vi "ToTable.vi"(8 "error in":errorcluster, 9 "Table Index (0)":i32, 10 "variant":variant, 11 "Sequencer Module editor node in":refnum<class "Sequencer Module editor node.lvclass">) -> (0 "error out":errorcluster, 1 "row headers":string[](array[string]), 2 "table":string[][](array[string]), 3 "Sequencer Module editor node out":refnum<class "Sequencer Module editor node.lvclass">)   [LabVIEW 2015, in "Sequencer Module editor node.lvclass"]
doc: "Generates the strings needed to display on a table based on the information found in the engine and module configuration classes."
uses:
  Sequencer Module editor node.lvclass
  module/configuration/Sequencer Module configuration.lvclass
  <vilib>/NI/Module Execution Interface/Engine Configuration/engine configuration.lvclass
  <vilib>/NI/DCAF/Tag Editor Core/control module/editor node/control module editor.lvclass
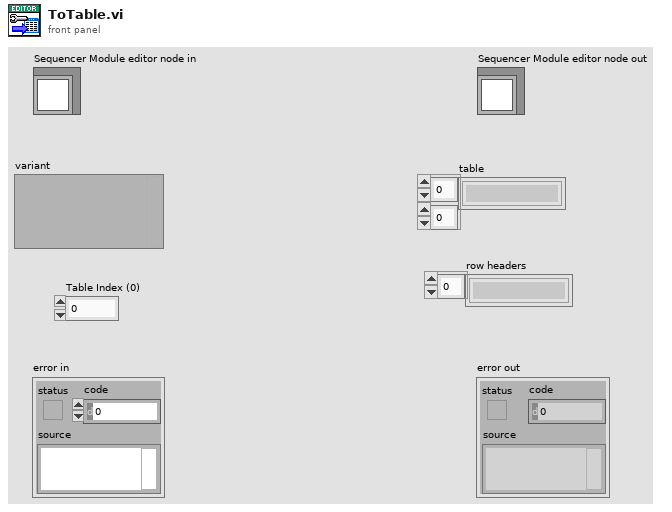
[diagram p1: front panel]
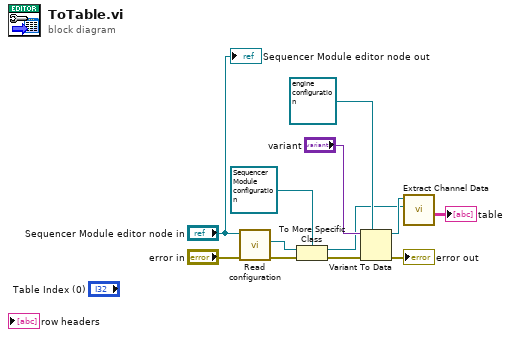
[diagram p0: block diagram]
diagram:
  n1 = call-dynamic "Read configuration.vi"("error in"="error in", "Sequencer Module editor node in"="Sequencer Module editor node in") -> ("error out"=w12:errorcluster, "configuration"=w6:refnum<class "NISE_CEF_serializable configuration.lvclass">)  [unwired: 7 in, 1 out]
  n2 = To More Specific Class(target class=refnum<class "Sequencer Module configuration.lvclass"> refnum ("tag bus configurable plugin module configuration"), reference=w6, error in=w12) -> (specific class reference=w2:refnum<class "Sequencer Module configuration.lvclass">, error out=w5:errorcluster)
  n3 = Variant To Data(error in=w5, type=refnum<class "engine configuration.lvclass"> refnum ("engine configuration"), Variant="variant") -> (data=w3:refnum<class "engine configuration.lvclass">, error out=→"error out":errorcluster)
  n4 = call <vilib>:"Extract Channel Data.vi"("module configuration in"=w2, "Engine Configuration"=w3) -> ("Channel Data"=→"table":string[][])  [unwired: 9 in]
  "Sequencer Module editor node out" <- "Sequencer Module editor node in"
